vi "X Array Range to Index.vi"(1 "X Range (data)":dbl, 2 "X-array":dbl[](array[numeric])) -> (0 "X Range (points)":i32)   [LabVIEW 2019, in "xy_utilities.lvlib"]
uses:
  xy_utilities.lvlib
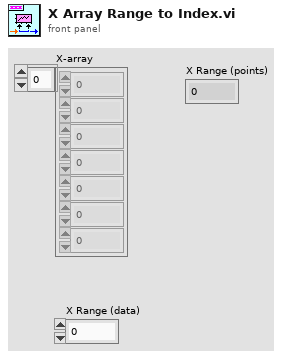
[diagram p1: front panel]
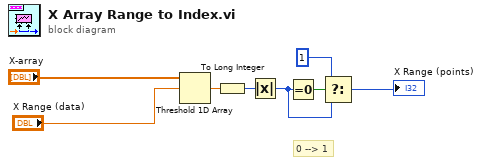
[diagram p0: block diagram]
diagram:
  # "0 --> 1"
  n1 = Threshold 1D Array(2:"X Range (data)", 3:"X-array") -> (0:w1:dbl)  [unwired: 1 in]
  n2 = To Long Integer(number=w1) -> (32bit integer=w8:i32)
  n3 = Absolute Value(x=w8) -> (abs(x)=w5:i32)
  n4 = Equal To 0?(x=w5) -> (x = 0?=w6:bool)
  n5 = Select(t=1, s=w6, f=w5) -> (s? t:f=→"X Range (points)":i32)
